vi "layout.vi"(0 "reference":refnum<class "NoteNode.lvclass">, 1 "graph":refnum<class "Graph.lvclass">, 2 "graphics":refnum<class "Graphics.lvclass">, 3 "grid":refnum<class "Grid.lvclass">, 5 "error in (no error)":errorcluster) -> (14 "reference out":refnum<class "NoteNode.lvclass">, 19 "error out":errorcluster)   [LabVIEW 2020, in "NoteNode.lvclass"]
doc: "public void layout(Graph g, Graphics2D g2, Grid grid)"
uses:
  <resource>/Framework/Providers/Open_GDS/UML/NoteNode_class/NoteNode.lvclass
  C:/Program Files (x86)/National Instruments/LabVIEW 2020/resource/Framework/Providers/Open_GDS/UML/RectangularNode_class/RectangularNode.lvclass
  <resource>/Framework/Providers/Open_GDS/UML/Graph_class/Graph.lvclass
  <resource>/Framework/Providers/Open_GDS/UML/Graphics_class/Graphics.lvclass
  <resource>/Framework/Providers/Open_GDS/UML/Grid_class/Grid.lvclass
  <resource>/Framework/Providers/Open_GDS/UML/MultiLineString_class/MultiLineString.lvclass
  <resource>/Framework/Providers/Open_GDS/UML/RectangularNode_class/RectangularNode.lvclass
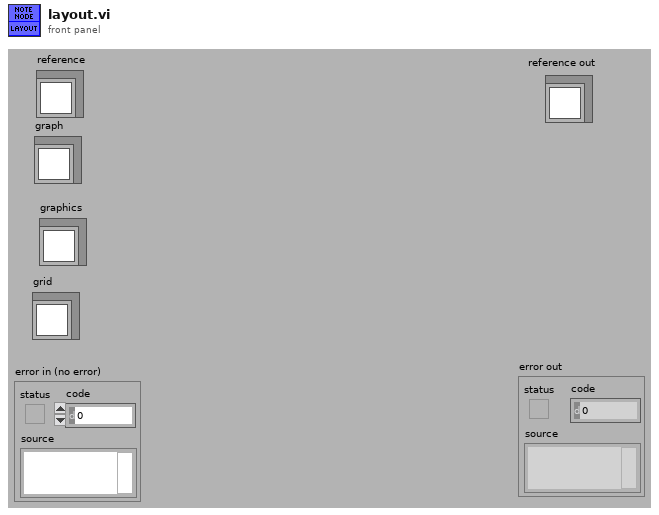
[diagram p1: front panel]
types:
  T1 = typedef "NoteNode.lvclass/ObjectAttributes.ctl" = cluster{"DEFAULT_WIDTH":i32, "DEFAULT_HEIGHT":i32, "DEFAULT_COLOR":u32, "FOLD_X":i32, "FOLD_Y":i32, "color":u32, "text":refnum<class "MultiLineString.lvclass">, "pointNodes":refnum<class "AbstractNode.lvclass">[]}
  T2 = typedef "RectangularNode.lvclass/ObjectAttributes.ctl" = cluster{"bounds":T3}
  T3 = typedef "Rectangle Rectangle2D.ctl" = cluster{"x":dbl, "y":dbl, "width":dbl, "height":dbl}
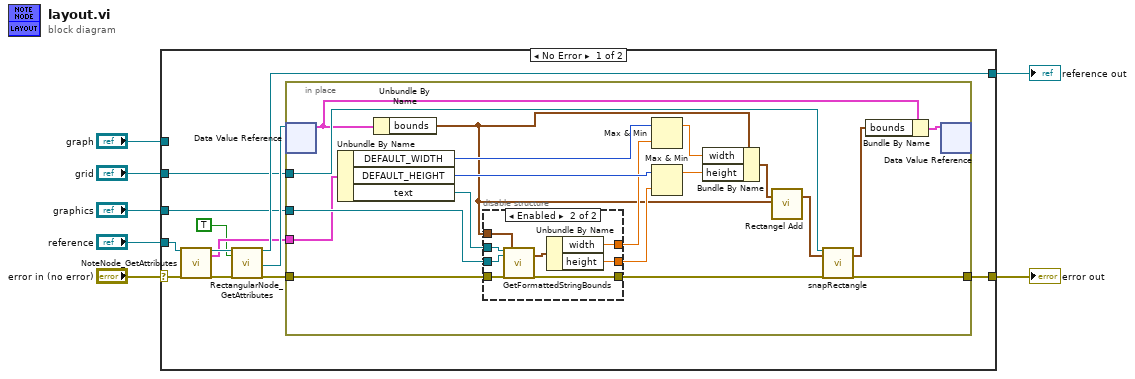
[diagram p0: block diagram]
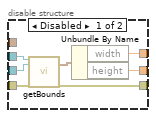
[diagram p2: hidden frame]
diagram:
  n1 = case shown="No Error" "error in (no error)" {
    selector: "error in (no error)" -> [w16 w54]
    tunnel: "reference" -> [w19 w55]
    tunnel: [w18 w54] -> w6
    tunnel: [w17 w55] -> w5
    tunnel: "graphics" -> [w12 _]
    tunnel: "grid" -> [w10 _]
    tunnel: "graph" -> [_ _]
    frame No Error {
      n2 = call <resource>:"NoteNode_GetAttributes.vi"("reference in"=w19, "error in (no error)"=w16) -> ("reference out"=w15:refnum<class "NoteNode.lvclass">, "Data"=w9:T1, "error out"=w14:errorcluster)  [unwired: 14 in, 1 out]
      n3 = call <resource>:"RectangularNode_GetAttributes.vi"("reference in"=w15, "OnlyGetDvrReference(False)"=TRUE, "error in (no error)"=w14) -> ("reference out"=w17:refnum<class "NoteNode.lvclass">, "DataRef"=w13:refnum<data-value>, "error out"=w11:errorcluster)  [unwired: 13 in, 1 out]
      n4 = in-place {
        in-place-border: w12 -> [w31]
        in-place-border: w11 -> [w30]
        in-place-border: w10 -> [w26]
        in-place-border: [w23] -> w18
        in-place-border: w9 -> [w20]
        n5 = in-place-dvr #1(w13) -> (w22:T2)  [unwired: 1 out]
        n6 = Unbundle By Name(w20) -> ("DEFAULT_WIDTH"=w38:i32, "DEFAULT_HEIGHT"=w37:i32, "text"=w36:refnum<class "MultiLineString.lvclass">)
        n7 = Unbundle By Name(w22) -> ("bounds"=w29:T3)
        n8 = disable-structure shown="Enabled" {
          disable-tunnel: w31 -> [w45 w52]
          disable-tunnel: w36 -> [w44 w53]
          disable-tunnel: w30 -> [w43 w51]
          disable-tunnel: [w41 w48] -> w35
          disable-tunnel: [w40 w47] -> w33
          disable-tunnel: [w39 w50] -> w28
          disable-tunnel: w29 -> [_ w46]
          frame Disabled {
            n9 = call-dynamic "getBounds.vi"("reference"=w44, "graphics"=w45, "error in (no error)"=w43) -> ("bounds"=w42:T3, "error out"=w39:errorcluster)  [unwired: 15 out]
            n10 = Unbundle By Name(w42) -> ("width"=w41:dbl, "height"=w40:dbl)
          }
          frame Enabled {
            n11 = call-dynamic "GetFormattedStringBounds.vi"("reference"=w53, "graphics"=w52, "error in (no error)"=w51, "TargetBounds(IgnoreIfZero)"=w46) -> ("bounds"=w49:T3, "error out"=w50:errorcluster)  [unwired: 13 in, 1 out]
            n12 = Unbundle By Name(w49) -> ("width"=w48:dbl, "height"=w47:dbl)
          }
        }
        n13 = Max & Min(x=w38, y=w35) -> (max(x,y)=w34:dbl)  [unwired: 1 out]
        n14 = Max & Min(x=w37, y=w33) -> (max(x,y)=w32:dbl)  [unwired: 1 out]
        n15 = Bundle By Name(cluster=w29, "width"=w34, "height"=w32) -> (w27:T3)
        n16 = call <resource>:"Rectangel Add.vi"("bounds1"=w27, "bounds2"=w29) -> ("boundsAdded"=w25:T3)  [unwired: 3 in, 14 out]
        n17 = call <resource>:"snapRectangle.vi"("reference"=w26, "bounds"=w25, "error in (no error)"=w28) -> ("boundsOut"=w24:T3, "error out"=w23:errorcluster)  [unwired: 15 out]
        n18 = Bundle By Name(cluster=w22, "bounds"=w24) -> (w21:T2)
        n19 = in-place-dvr #1(w21) -> ()  [unwired: 2 out]
      }
    }
    frame Error {
    }
  }
  "reference out" <- w5
  "error out" <- w6
